vi "LSCI332 SetRelayOutput.vi"(0 "VISA Rsrc":refnum<visa-resource-name>="GPIB0::12::INSTR", 5 "Relay(1)":u32(ring) caption="Relay" items=["Relay 1", "Relay 2"], 7 "RelayMode":enum16{"Off", "On", "Alarm"}(ring) caption="Relay Mode", 9 "Alarm Input":enum16{"A", "B"}(ring), 11 "error in":errorcluster, 12 "Alarm Type":enum16{"Low", "High", "Low&High"}(ring)) -> (15 "error out":errorcluster)   [LabVIEW 2019]
doc: "Ce Vi envoie à l'instrument la valeur de \"Manual output\" de chauffage désiré, en %."
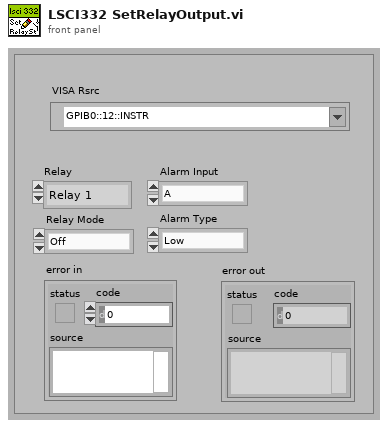
[diagram p1: front panel]
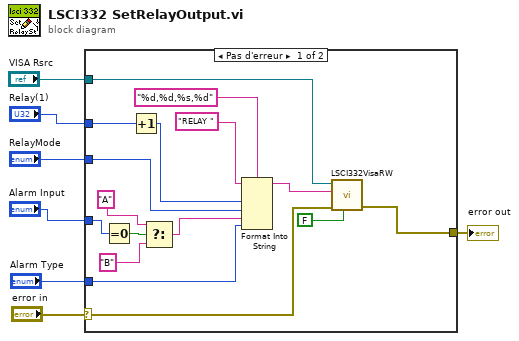
[diagram p0: block diagram]
diagram:
  n1 = case shown="Pas d'erreur" "error in" {
    selector: "error in" -> [w22 w24]
    tunnel: [w19 w24] -> w7
    tunnel: "VISA Rsrc" -> [w23 _]
    tunnel: "Relay(1)" -> [w18 _]
    tunnel: "RelayMode" -> [w14 _]
    tunnel: "Alarm Input" -> [w13 _]
    tunnel: "Alarm Type" -> [w8 _]
    frame No Error {
      n2 = Equal To 0?(x=w13) -> (x = 0?=w12:bool)
      n3 = Increment(x=w18) -> (x+1=w15:u32)
      n4 = Select(t="A", s=w12, f="B") -> (s? t:f=w9:string)
      n5 = Format Into String(format string="%d,%d,%s,%d", initial string="RELAY ", w15, w14, w9, w8) -> (resulting string=w16:string)  [unwired: 1 in, 1 out]
      n6 = call <userlib>:"LSCI332VisaRW.vi"("Lecture?(T)"=FALSE, "error in (no error)"=w22, "ChaineCom"=w16, "VISA Rsrc"=w23) -> ("error out"=w19:errorcluster)  [unwired: 3 in, 3 out]
    }
    frame Error {
    }
  }
  "error out" <- w7
